vi "Delta.vi"(10 "Initial Input":dbl, 11 "Data":dbl) -> (3 "Delta":dbl)   [LabVIEW 2015]
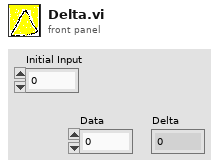
[diagram p1: front panel]
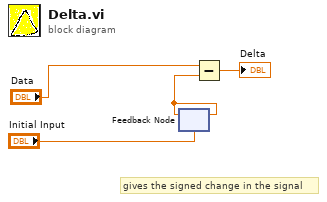
[diagram p0: block diagram]
diagram:
  # "gives the signed change in the signal"
  n1 = feedback #1("Initial Input") -> (w2:dbl)
  n2 = feedback-in #1(w2) -> ()
  n3 = Subtract(x="Data", y=w2) -> (x-y=→"Delta":dbl)
